vi "ToPath.vi"(8 "error in":errorcluster, 11 "Path in":refnum<class "Generic.lvclass">) -> (0 "error out":errorcluster, 3 "Path out":refnum<class "Path.lvclass">)   [LabVIEW 2014, in "Path.lvclass"]
uses:
  Path.lvclass
  Generic/Generic.lvclass
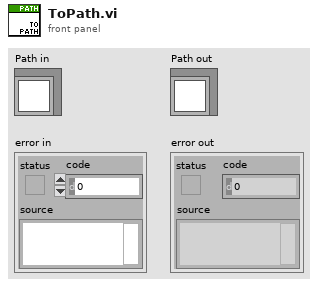
[diagram p1: front panel]
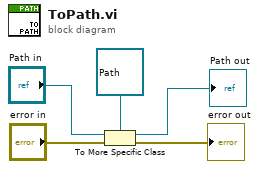
[diagram p0: block diagram]
diagram:
  n1 = To More Specific Class(target class=refnum<class "Path.lvclass"> refnum ("Path in"), reference="Path in", error in="error in") -> (specific class reference=→"Path out":refnum<class "Path.lvclass">, error out=→"error out":errorcluster)
